vi "Th_GUI.vi"() -> ()   [LabVIEW 2018]
panel:
  in  "?":bool
  in  "?":bool
  in  "3":bool
  in  "Light":bool
  in  "Lap RESET":bool
  in  "Lap":bool
  in  "seconds":dbl
  in  "minutes":dbl
  in  "hour":dbl
  in  "Power":bool
  in  "Mode":string(combo)
  in  "Time":dbl format="%<%H:%M:%S%3u>t"
  in  "START":bool
  in  "LapTime":dbl[](array[numeric]) format="%<%H:%M:%S%3u>t"
  in  "RESET":bool
  in  "STOP":bool
  out "現在時刻":dbl
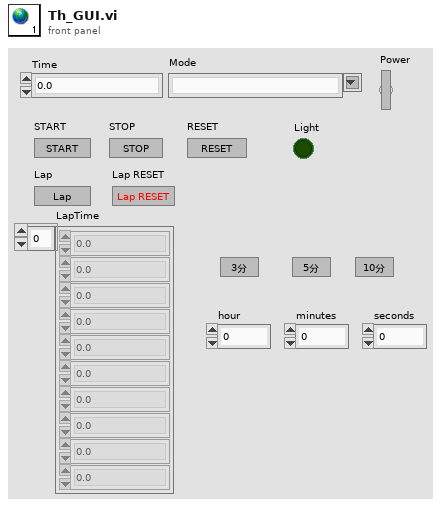
[diagram p1: front panel]
diagram:
